vi "pruebas con PQ Alarma Log.vi"() -> ()   [LabVIEW 2018]
panel:
  out "Array":sgl[][](array[numeric])
  in  "Descending (F)":bool
  out "PQ_Log array out 4":sgl[][](array[numeric])
  out "Numeric":i32
  out "PQ_Log array out":sgl[](array[numeric])
  out "PowerQualityLog out":T1
  out "Boolean array 6":bool[](array[boolean])
  in  "stop":bool
  # "Sag_Indication_Detected"
  # "Swell_Indication_Detected"
  # "Transient_Indication"
  # "200mS_Sag_Swell_Status_Flag"
  # "3s_Sag_Swell_Status_Flag"
  # "10m_Sag_Swell_Status_Flag"
  # "2h_Sag_Swell_Status_Flag"
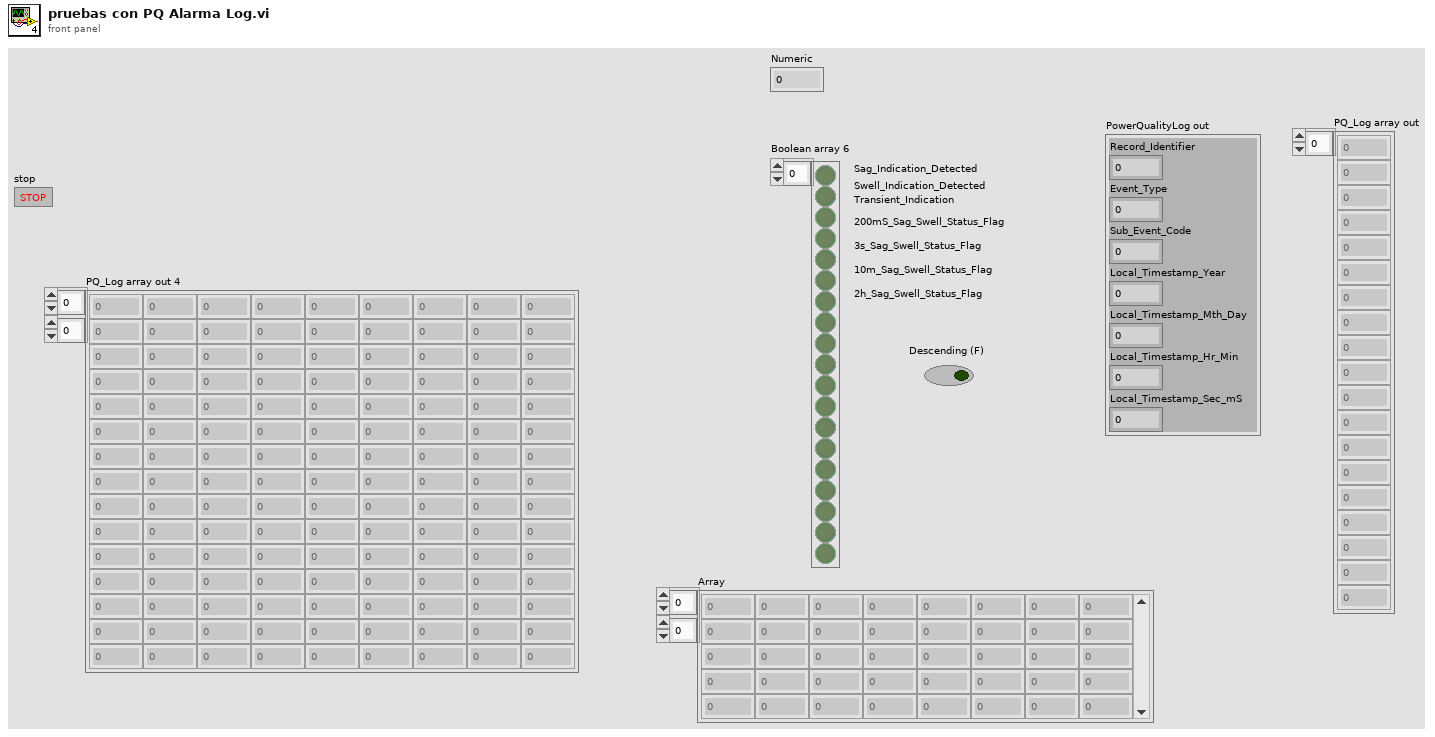
[diagram p1: front panel]
types:
  T1 = cluster{"Record_Identifier":sgl, "Event_Type":sgl, "Sub_Event_Code":sgl, "Local_Timestamp_Year":sgl, "Local_Timestamp_Mth_Day":sgl, "Local_Timestamp_Hr_Min":sgl, "Local_Timestamp_Sec_mS":sgl}
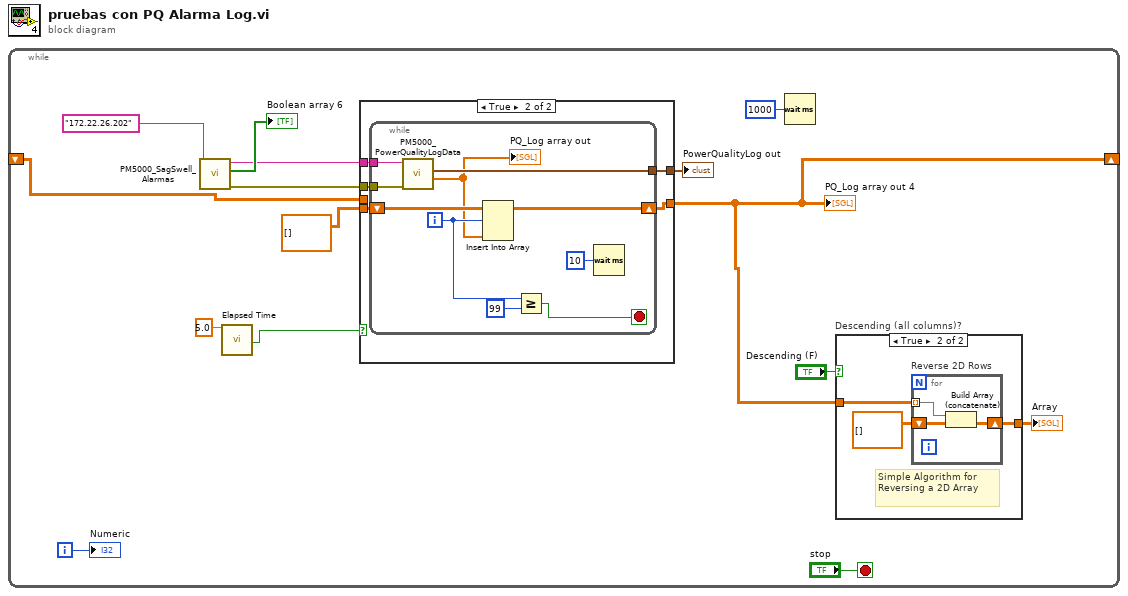
[diagram p0: block diagram]
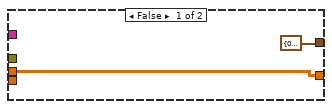
[diagram p3: hidden frame]
diagram:
  n1 = while {
    shift-right: [w2] -> _
    shift-left: _ -> [w4]
    i -> [w8]
    stop <- "stop" stop-if-true
    n2 = call "PM5000_SagSwell_Alarmas.vi"("Network Path"="172.22.26.202") -> ("error out"=w10:errorcluster, "PQ_Alarmas"=→"Boolean array 6":bool[], "Network Path out"=w11:string)  [unwired: 8 in]
    n3 = call "Elapsed Time"("Time Target (s)"=5.0) -> ("Time has Elapsed"=w5:bool)  [unwired: 11 in, 7 out]
    n4 = case shown="True" w5 {
      tunnel: w11 -> [_ w29]
      tunnel: w10 -> [_ w28]
      tunnel: [T1 {"Record_Identifier"=0.0, "Event_Type"=0.0, "Sub_Event_Code"=0.0, "Local_Timestamp_Year"=0.0, "Local_Timestamp_Mth_Day"=0.0, "Local_Timestamp_Hr_Min"=0.0, "Local_Timestamp_Sec_mS"=0.0} ("PowerQualityLog out") w27] -> w9
      tunnel: sgl[][] [] -> [_ w26]
      tunnel: [w24 w25] -> w2
      tunnel: w4 -> [w24 _]
      frame False {
      }
      frame True {
        n5 = while {
          tunnel: w29 -> [w39]
          tunnel: w28 -> [w38]
          tunnel: [w37] -> w27
          shift-right: [w35] -> w25
          shift-left: w26 -> [w36]
          i -> [w34]
          stop <- w32 stop-if-true
          n6 = call "PM5000_PowerQualityLogData.vi"("error in"=w38, "Network Path"=w39) -> ("PQ_Log array out"=w31:sgl[], "PowerQualityLog out"=w37:T1)  [unwired: 6 in, 2 out]
          "PQ_Log array out" <- w31
          n7 = Insert Into Array(array=w36, index (row)=w34, new element=w31) -> (w35:sgl[][])  [unwired: 1 in]
          n8 = Greater Or Equal?(x=w34, y=99) -> (x >= y?=w32:bool)
          n9 = Wait (ms)(milliseconds to wait=u32 10) -> ()  [unwired: 1 out]
        }
      }
    }
    "PowerQualityLog out" <- w9
    "PQ_Log array out 4" <- w2
    n10 = Wait (ms)(milliseconds to wait=u32 1000) -> ()  [unwired: 1 out]
    n11 = case "Descending (all columns)?" shown="True" "Descending (F)" {
      tunnel: w2 -> [w16 w18]
      tunnel: [w16 w17] -> w1
      frame False {
      }
      frame True {
        # "Simple Algorithm for Reversing a 2D Array"
        n12 = for "Reverse 2D Rows" {
          tunnel: w18 -> [w22] mode=indexing
          shift-right: [w20] -> w17
          shift-left: sgl[][] [] -> [w21]
          n13 = Build Array (concatenate)(w22, w21) -> (w20:sgl[][])
        }
      }
    }
    "Array" <- w1
    "Numeric" <- w8
  }
